vi "merFISH_define_injections_procedure.vi"(0 "Injection procedure IN photobleaching":i32[][](array[numeric]), 1 "Injection procedure IN hybridization":i32[][](array[numeric]), 5 "Buffer Refnum":refnum<vi>, 9 "Start acquisition":bool, 11 "error in":errorcluster, 12 "Defaut injection":i32[][](array[numeric])=[[10, 500, 350, 0], [0, 1200, 120, 0], [10, 500, 300, 21], [5, 2000, 222, 21], [10, 1200, 300, 22], [5, 800, 350, 1], [0, 150, 100, 1]], 13 "Defaut injection photobleaching":i32[][](array[numeric])=[[10, 500, 350, 0], [0, 1200, 120, 0], [10, 500, 300, 21], [5, 2000, 222, 21], [10, 1200, 300, 22], [5, 800, 350, 1], [0, 150, 100, 1]]) -> (3 "Injection procedure OUT":i32[][](array[numeric]), 4 "Injection procedure OUT\nPhotobleaching":i32[][](array[numeric]), 6 "Next task":T1, 10 "error out":errorcluster, 14 "Item Names photobleaching":string[](array[string]), 15 "Item Names":string[](array[string]))   [LabVIEW 2015]
uses:
  CONTROLS/Q_main_element.ctl
panel:
  in  "Default":bool
  in  "Flow rate (µl/min)":i32
  in  "Remove photobleaching":bool
  in  "Select application":i32(ring) caption="Select procedure application" items=["Select procedure application", "HYBRIDIZATION", "PHOTOBLEACHING"]
  in  "Injection procedure PHOTOBLEACHING":i32(listbox)=-1
  in  "Volume (µl)":i32
  in  "Remove":bool
  in  "stop":bool
  in  "Injection procedure HYBRIDIZATION":i32(listbox)=-1
  in  "Add":bool
  in  "Select product":i32(ring) items=["Select product to inject", "ssc", "wb", "ib", "merFISH probe"]
  in  "Pressure (mbar)":i32
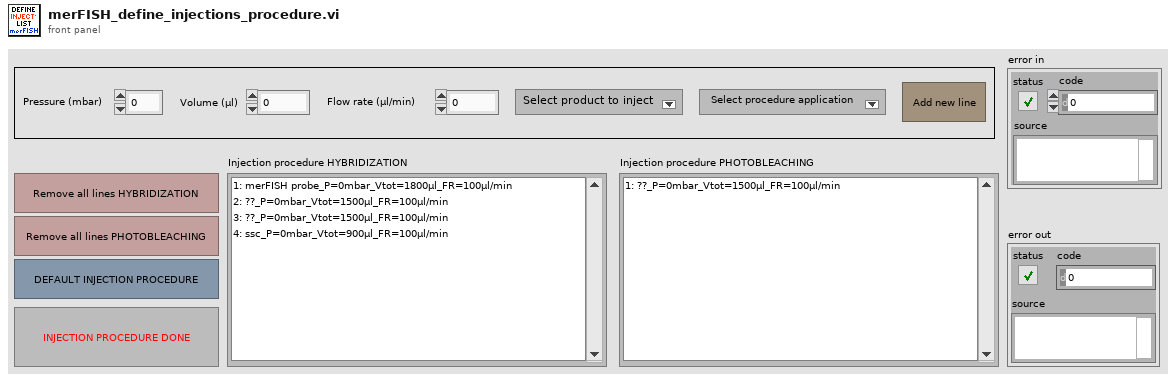
[diagram p1: front panel]
types:
  T1 = typedef "Q_main_element.ctl" = cluster{"variant":variant, "Instruction":enum16{"Main_idle", "Main_initialize", "Main_initialize_TDMS", "Main_initialize_Queue", "Main_error", "Main_DAQ_initialization_results", "Main_ASI_initialization_results", "Main_Piezo_initialization_results", "Main_Valve_initialization_results", "Main_Pump_initialization_results", "Main_CAMERA_initialization_results", "Main_FPGA_initialization_results", "Main_DAQ_error", "Main_ASI_error", "Main_Piezo_error", "Main_CAMERA_error", "Main_Valve_error", "Main_Pump_error", "Main_FPGA_error", "Main_start_acquiring", "Main_not_acquiring", "Main_acquiring", "Main_stop_acquiring", "Main_change_exposure", "Main_change_z_scan_parameters", "Main_define_ROI", "Main_define_mosaic", "Main_read_kinetic_time", "Main_cooler", "Main_read_temperature", "Main_save_XY", "Main_load_XY", "Main_discard_XY", "Main_move_to_XY", "Main_measure_QPD", "Main_autofocus_calibration", "Main_autofocus_initialization", "Main_autofocus_stop", "Main_save_PID", "Main_change_H_valve_position", "Main_two_way_valve", "Main_save_movie", "Main_init_single_scan", "Main_single_scan", "Main_stop_single_scan", "Main_merFISH_illumination_parameters", "Main_merFISH_buffer_probe_list", "Main_merFISH_injections_procedure", "Main_merFISH_save_setpoint", "Main_merFISH_DAPI_parameters", "Main_merFISH_Brightfield_parameters", "Main_merFISH_save_embryo_ROI", "Main_merFISH_init", "Main_merFISH_resume", "Main_merFISH_start_autofocus", "Main_merFISH_open_close_valve_merFISH", "Main_merFISH_open_close_valve_photobleaching", "Main_merFISH_hybridization", "Main_merFISH_move_to_ROI", "Main_merFISH_wait_stabilization", "Main_merFISH_move_to_REF", "Main_merFISH_scan", "Main_merFISH_photobleaching_injection", "Main_merFISH_photobleaching", "Main_merFISH_send_email", "Main_merFISH_close", "Main_STOP"}}
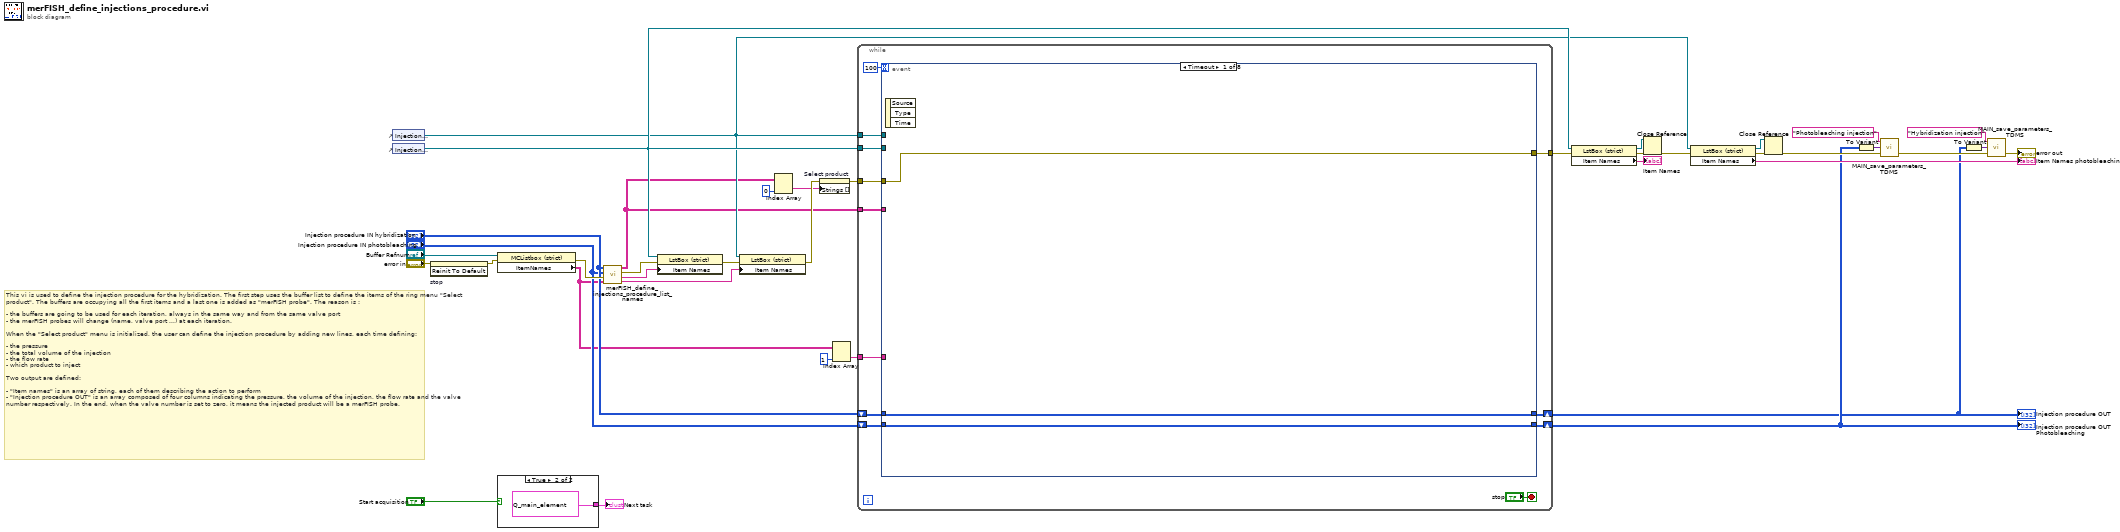
[diagram p0: block diagram]
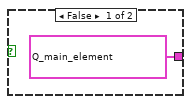
[diagram p2: hidden frame]
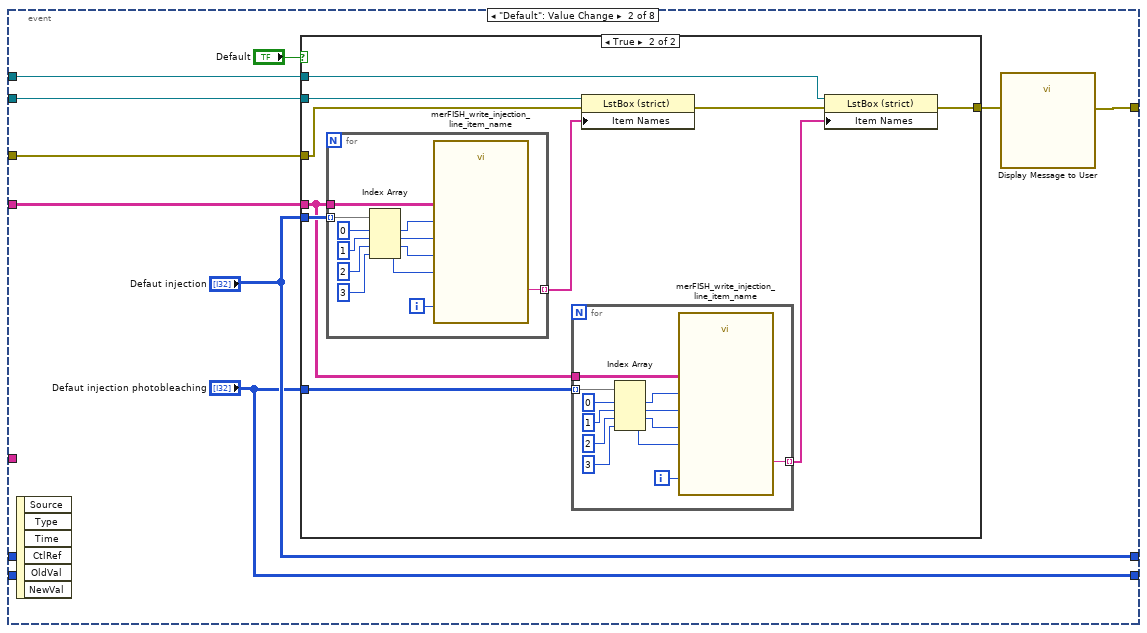
[diagram p3: hidden frame]
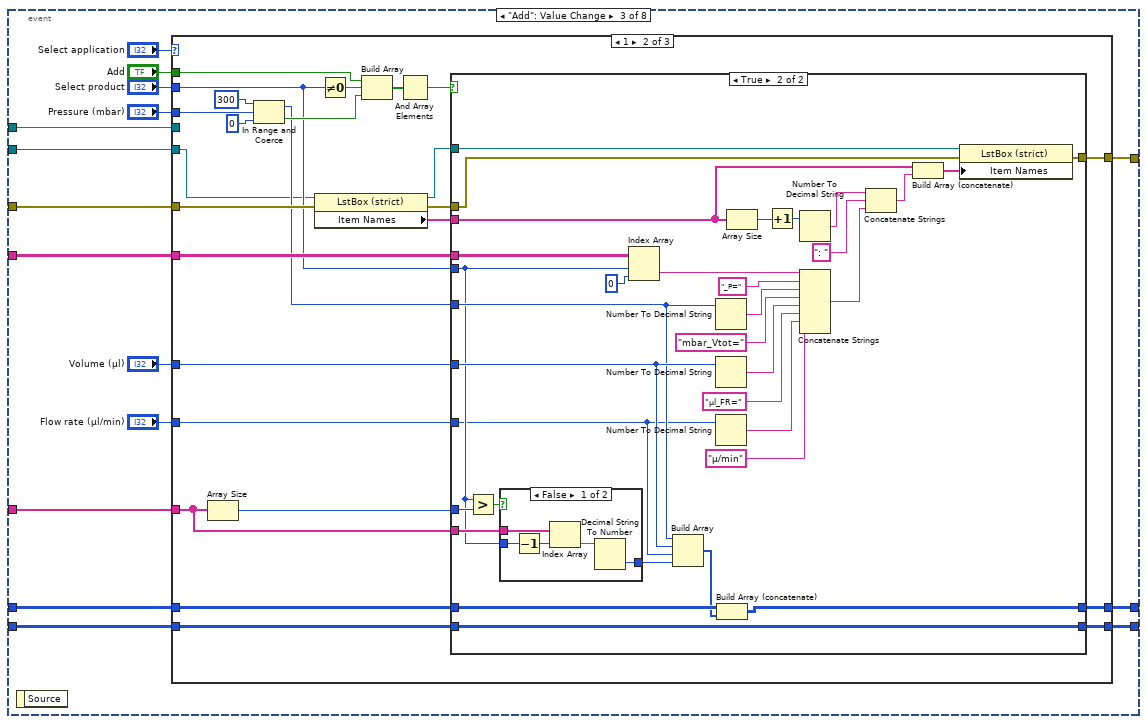
[diagram p5: hidden frame]
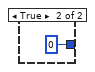
[diagram p8: hidden frame]
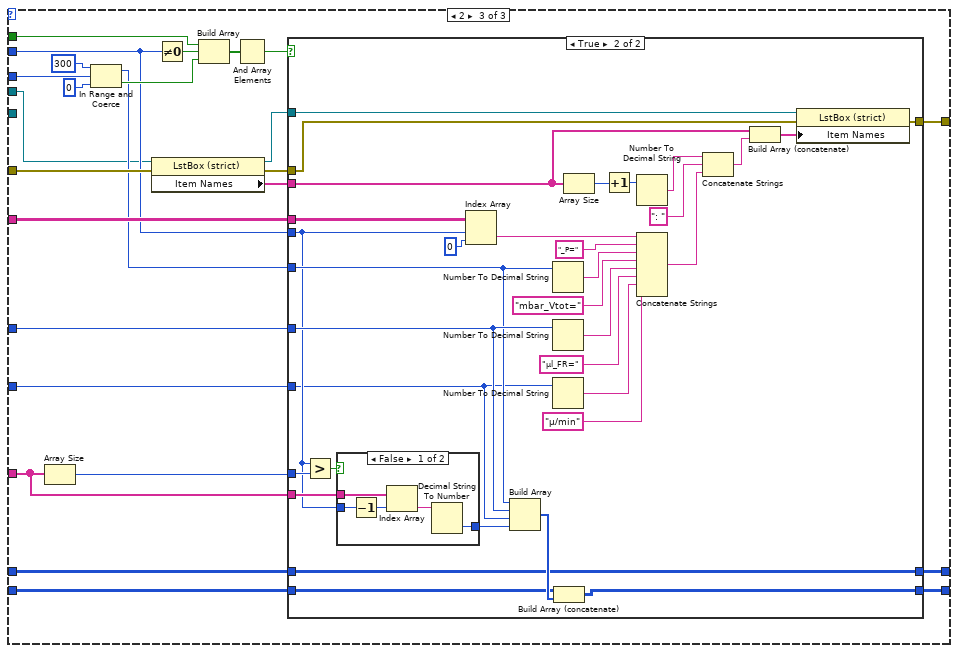
[diagram p9: hidden frame]
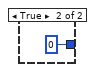
[diagram p11: hidden frame]
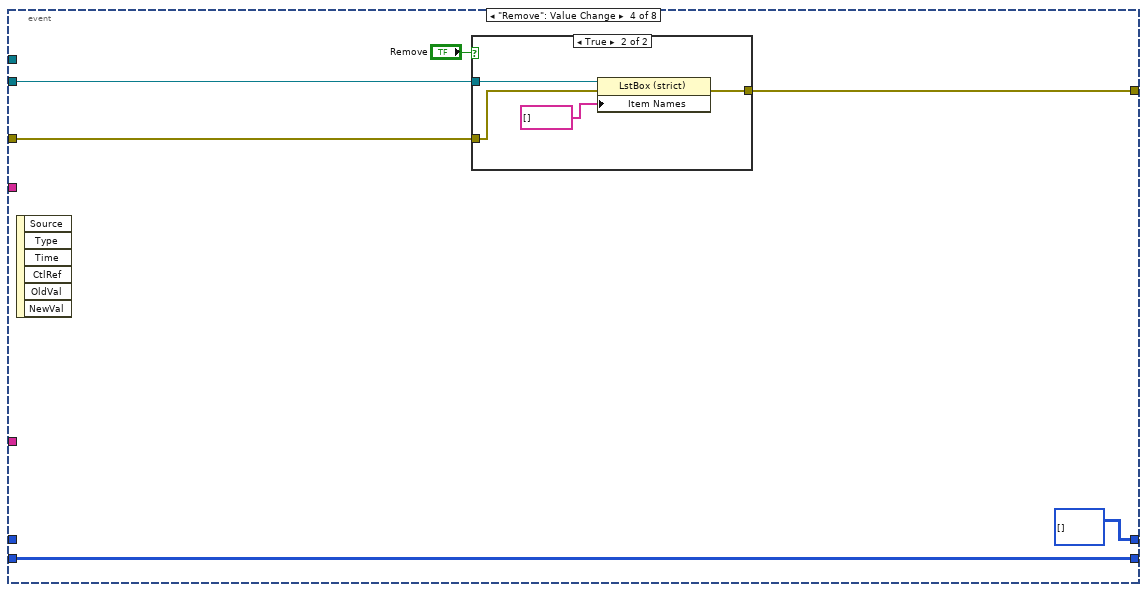
[diagram p12: hidden frame]
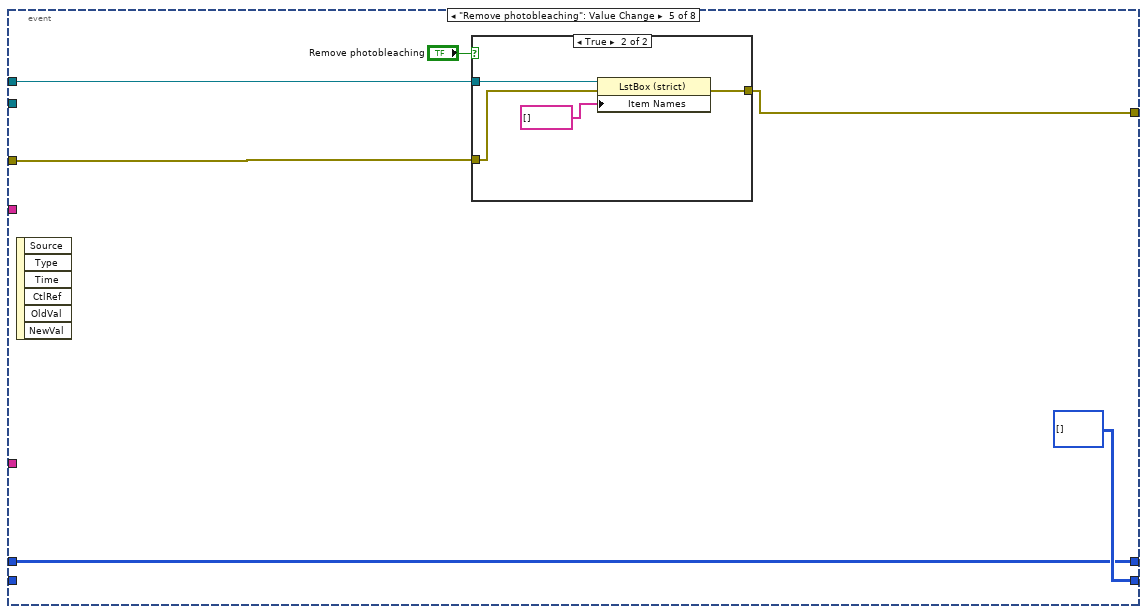
[diagram p14: hidden frame]
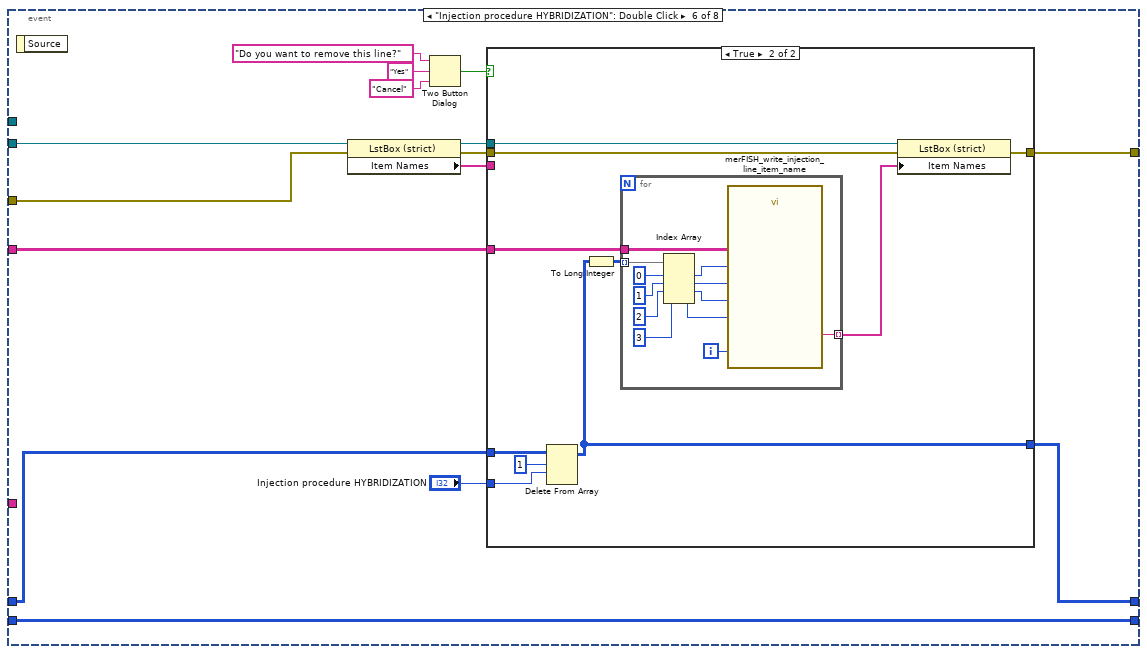
[diagram p16: hidden frame]
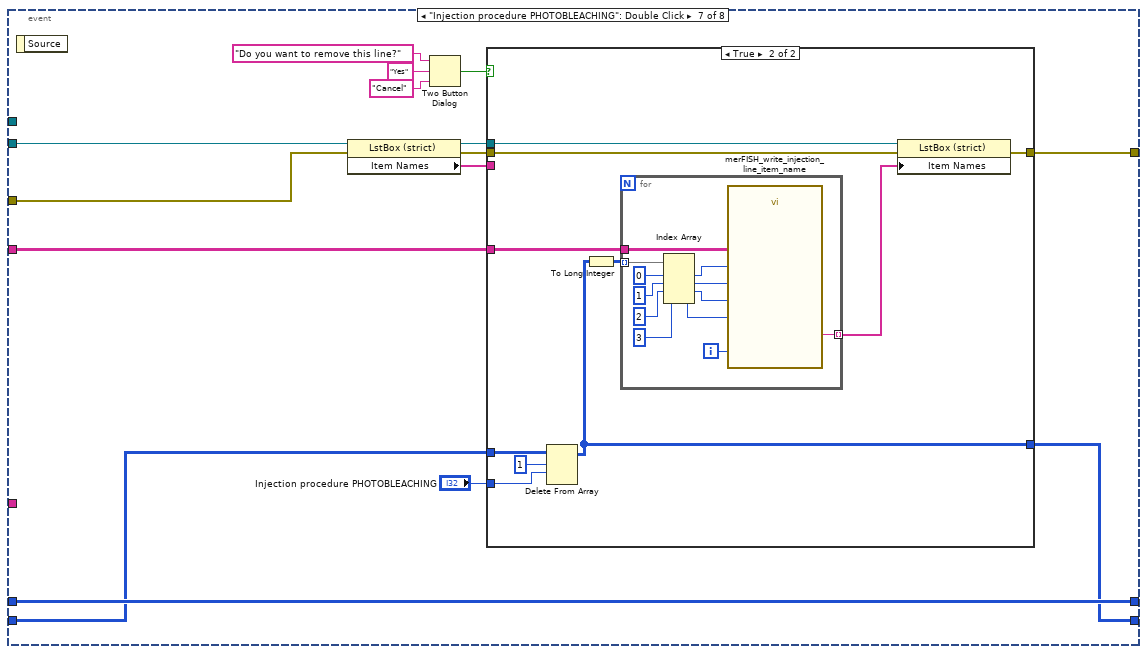
[diagram p18: hidden frame]
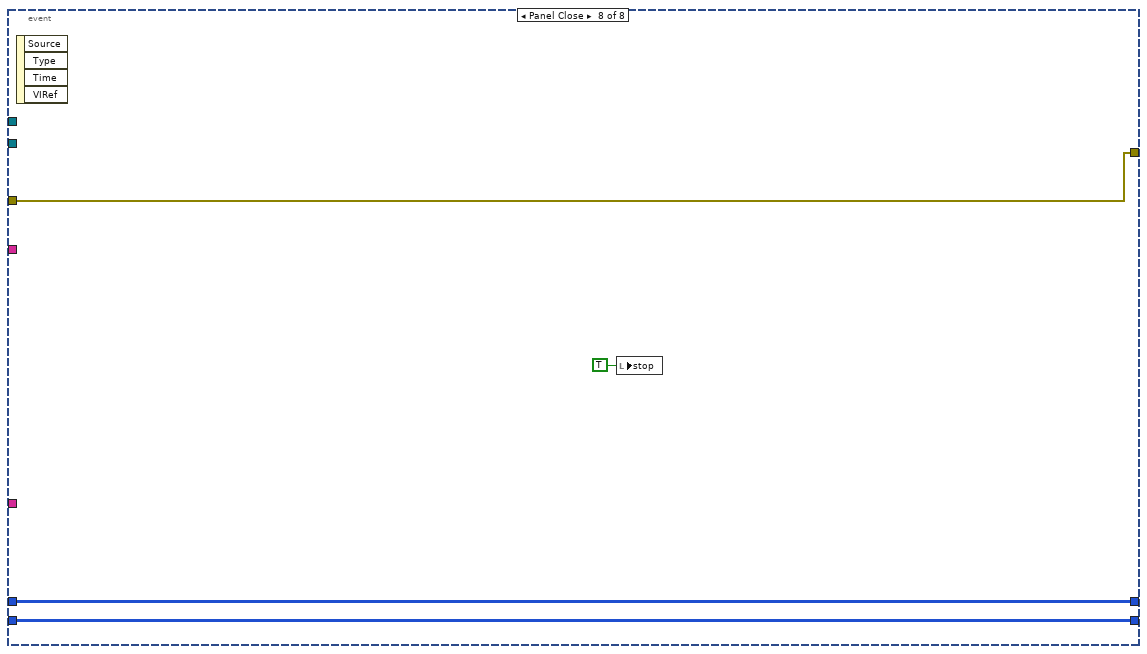
[diagram p20: hidden frame]
diagram:
  # "This vi is used to define the injection procedure for the hybridization. The first step uses the buffer list to define the items of the ring menu \"Select product\". The buffers are occupying all the first items and a last one is added as \"merFISH probe\". The reason is :\n\n- the buffers are going to be used for each iteration, always in the same way and from the same valve port\n- the merFISH probes will change (name, valve port ...) at each iteration.\n\nWhen the \"Select product\" menu is initialized, the user can define the injection procedure by adding new lines, each time defining:\n\n- the pressure\n- the total volume of the injection\n- the flow rate\n- which product to inject\n\nTwo output are defined:\n\n- \"Item names\" is an array of string, each of them describing the action to perform\n- \"Injection procedure OUT\" is an array composed of four columns indicating the pressure, the volume of the injection, the flow rate and the valve number respectively. In the end, when the valve number is set to zero, it means the injected product will be a merFISH probe."
  n1 = control-ref of="Injection procedure PHOTOBLEACHING"() -> (w29:refnum<vi>)
  n2 = control-ref of="Injection manager"() -> (w38:refnum<vi>)
  n3 = invoke on="stop" class="Bool (strict)" method="Reinit To Default"(error in="error in") -> (error out=w1:errorcluster)  [unwired: 2 in, 2 out]
  n4 = property class="MCListbox (strict)"(reference="Buffer Refnum", error in=w1) -> (error out=w28:errorcluster, "ItemNames"=w22:string[][])  [unwired: 1 out]
  n5 = case shown="True" "Start acquisition" {
    tunnel: [T1 {"variant"=variant, "Instruction"=enum."Main_not_acquiring"} ("Q_main_element") T1 {"variant"=variant, "Instruction"=enum."Main_acquiring"} ("Q_main_element")] -> w12
    frame False {
    }
    frame True {
    }
  }
  "Next task" <- w12
  n6 = call "merFISH_define_injections_procedure_list_names.vi"("Buffer list"=w22, "error in"=w28, "Injection procedure IN photobleaching"="Injection procedure IN photobleaching", "Injection procedure IN hybridization"="Injection procedure IN hybridization") -> ("Photobleaching name"=w25:string[], "Hybridization name"=w26:string[], "error out"=w27:errorcluster, "Buffer selection list"=w19:string[][])
  n7 = property class="LstBox (strict)"(reference=w38, error in=w27, "Item Names"=w26) -> (error out=w33:errorcluster)  [unwired: 1 out]
  n8 = property class="LstBox (strict)"(reference=w29, error in=w33, "Item Names"=w25) -> (error out=w32:errorcluster)  [unwired: 1 out]
  n9 = Index Array(array=w19, index (col)=0 ("index (row)")) -> (element=w20:string[])  [unwired: 1 in]
  n10 = property on="Select product" class="Ring (strict)"(error in=w32, "Strings []"=w20) -> (error out=w37:errorcluster)  [unwired: 1 in, 1 out]
  n11 = Index Array(array=w22, index (col)=1 ("disabled index (col)")) -> (element=w34:string[])  [unwired: 1 in]
  n12 = while {
    tunnel: w38 -> [w51]
    tunnel: [w50] -> w39
    tunnel: w19 -> [w49]
    shift-right: [w47] -> w3
    shift-left: "Injection procedure IN hybridization" -> [w48]
    tunnel: w34 -> [w46]
    tunnel: w37 -> [w45]
    tunnel: w29 -> [w44]
    shift-right: [w42] -> w4
    shift-left: "Injection procedure IN photobleaching" -> [w43]
    stop <- "stop" stop-if-true
    n13 = event shown="[0] Timeout" {
      selector: _ -> [_ _ _ _ _ _ _ _]
      dyn-events: _ -> [_ _ _ _ _ _ _ _]
      timeout: 100 -> [_ _ _ _ _ _ _ _]
      tunnel: w51 -> [_ w64 w105 w259 _ w283 w324 _]
      tunnel: w45 -> [w56 w61 w114 w257 w270 w281 w322 w357]
      tunnel: [w56 w62 w116 w256 w269 w286 w325 w357] -> w50
      tunnel: w48 -> [w55 _ w115 _ w265 w285 w317 w356]
      tunnel: w49 -> [_ w65 w113 _ _ w277 w319 _]
      tunnel: [w55 "Defaut injection" w112 i32[][] [] ("Injection procedure IN") w265 w278 w317 w356] -> w47
      tunnel: w46 -> [_ _ w111 _ _ _ _ _]
      tunnel: w44 -> [_ w60 w106 _ w267 _ _ _]
      tunnel: w43 -> [w54 _ w104 w254 _ w276 w316 w355]
      tunnel: [w54 "Defaut injection photobleaching" w103 w254 i32[][] [] ("Injection procedure IN") w276 w315 w355] -> w42
      event Timeout {
        n14 = event-data() -> ()  [unwired: 1 in, 3 out]
      }
      event "Default": Value Change {
        n15 = event-data() -> ()  [unwired: 1 in, 6 out]
        n16 = case shown="True" "Default" {
          tunnel: w65 -> [_ w71]
          tunnel: w64 -> [_ w76]
          tunnel: [w66 w69] -> w63
          tunnel: "Defaut injection" -> [_ w74]
          tunnel: w61 -> [w66 w73]
          tunnel: w60 -> [_ w67]
          tunnel: "Defaut injection photobleaching" -> [_ w72]
          frame False {
          }
          frame True {
            n17 = for {
              tunnel: w74 -> [w99] mode=indexing
              tunnel: [w100] -> w75 mode=indexing
              tunnel: w71 -> [w95]
              i -> [w94]
              n18 = Index Array(array=w99, index #1=0 ("index"), index #2=1 ("index"), index #3=2 ("index"), index #4=3 ("index")) -> (element #1=w93:i32, element #2=w92:i32, element #3=w90:i32, element #4=w89:i32)
              n19 = call "merFISH_write_injection_line_item_name.vi"("Flow rate (µl/min)"=w90, "Select product"=w89, "Injection line number"=w94, "Buffer list"=w95, "Volume (µl)"=w92, "Pressure (mbar)"=w93) -> ("Task name"=w100:string)  [unwired: 3 in]
            }
            n20 = for {
              tunnel: w72 -> [w87] mode=indexing
              tunnel: [w88] -> w68 mode=indexing
              tunnel: w71 -> [w83]
              i -> [w82]
              n21 = Index Array(array=w87, index #1=0 ("index"), index #2=1 ("index"), index #3=2 ("index"), index #4=3 ("index")) -> (element #1=w81:i32, element #2=w80:i32, element #3=w78:i32, element #4=w77:i32)
              n22 = call "merFISH_write_injection_line_item_name.vi"("Flow rate (µl/min)"=w78, "Select product"=w77, "Injection line number"=w82, "Buffer list"=w83, "Volume (µl)"=w80, "Pressure (mbar)"=w81) -> ("Task name"=w88:string)  [unwired: 3 in]
            }
            n23 = property class="LstBox (strict)"(reference=w76, error in=w73, "Item Names"=w75) -> (error out=w70:errorcluster)  [unwired: 1 out]
            n24 = property class="LstBox (strict)"(reference=w67, error in=w70, "Item Names"=w68) -> (error out=w69:errorcluster)  [unwired: 1 out]
          }
        }
        n25 = call "Display Message to User"("error in (no error)"=w63) -> ("error out"=w62:errorcluster)  [unwired: 9 in, 1 out]
      }
      event "Add": Value Change {
        n26 = event-data() -> ()  [unwired: 1 in, 1 out]
        n27 = case shown="1" "Select application" {
          tunnel: [w118 w144 w211] -> w116
          tunnel: w115 -> [w119 w143 w210]
          tunnel: w114 -> [w118 w142 w209]
          tunnel: w113 -> [_ w132 w199]
          tunnel: [w119 w130 w197] -> w112
          tunnel: w111 -> [_ w128 w195]
          tunnel: "Add" -> [_ w127 w194]
          tunnel: "Select product" -> [_ w126 w193]
          tunnel: "Pressure (mbar)" -> [_ w125 w192]
          tunnel: w106 -> [_ _ w187]
          tunnel: w105 -> [_ w124 _]
          tunnel: w104 -> [w117 w123 w191]
          tunnel: [w117 w122 w190] -> w103
          tunnel: "Volume (µl)" -> [_ w121 w189]
          tunnel: "Flow rate (µl/min)" -> [_ w120 w188]
          frame 0, Default {
          }
          frame 1 {
            n28 = Array Size(array=w128) -> (size(s)=w129:i32)
            n29 = In Range and Coerce(upper limit=300, x=w125, lower limit=0) -> (coerced(x)=w131:i32, In Range?=w133:bool)
            n30 = property class="LstBox (strict)"(reference=w124, error in=w142) -> (reference out=w137:refnum<vi>, error out=w138:errorcluster, "Item Names"=w136:string[])
            n31 = Not Equal To 0?(x=w126) -> (x != 0?=w141:bool)
            n32 = Build Array(w127, w141, w133) -> (w140:bool[])
            n33 = And Array Elements(Boolean array=w140) -> (logical AND=w139:bool)
            n34 = case shown="True" w139 {
              tunnel: w137 -> [_ w177]
              tunnel: w126 -> [_ w156]
              tunnel: [w147 w173] -> w144
              tunnel: w138 -> [w147 w168]
              tunnel: w143 -> [w146 w172]
              tunnel: [w146 w171] -> w130
              tunnel: w136 -> [_ w169]
              tunnel: w121 -> [_ w161]
              tunnel: w132 -> [_ w167]
              tunnel: w131 -> [_ w159]
              tunnel: w129 -> [_ w158]
              tunnel: w128 -> [_ w157]
              tunnel: w123 -> [w145 w153]
              tunnel: [w145 w153] -> w122
              tunnel: w120 -> [_ w150]
              frame False {
              }
              frame True {
                n35 = Greater?(x=w156, y=w158) -> (0:w154:bool)
                n36 = case shown="False" w154 {
                  tunnel: w157 -> [w185 _]
                  tunnel: w156 -> [w184 _]
                  tunnel: [w181 0] -> w149
                  frame False {
                    n37 = Decrement(x=w184) -> (x-1=w183:i32)
                    n38 = Index Array(array=w185, index=w183) -> (element=w182:string)
                    n39 = Decimal String To Number(string=w182) -> (number=w181:i32)  [unwired: 2 in, 1 out]
                  }
                  frame True {
                  }
                }
                n40 = Index Array(array=w167, index (row)=w156, index (col)=0 ("disabled index (col)")) -> (element=w166:string)
                n41 = Build Array(w159, w161, w150, w149) -> (w155:i32[])
                n42 = Number To Decimal String(number=w159) -> (decimal integer string=w164:string)  [unwired: 1 in]
                n43 = Number To Decimal String(number=w161) -> (decimal integer string=w162:string)  [unwired: 1 in]
                n44 = Number To Decimal String(number=w150) -> (decimal integer string=w152:string)  [unwired: 1 in]
                n45 = Build Array (concatenate)(w172, w155) -> (w171:i32[][])
                n46 = Array Size(array=w169) -> (size(s)=w176:i32)
                n47 = Increment(x=w176) -> (x+1=w180:i32)
                n48 = Number To Decimal String(number=w180) -> (decimal integer string=w179:string)  [unwired: 1 in]
                n49 = Concatenate Strings(w166, "_P=" ("string"), w164, "mbar_Vtot=" ("string"), w162, "µl_FR=" ("string"), w152, "µ/min" ("string")) -> (w174:string)
                n50 = Concatenate Strings(w179, ": " ("string"), w174) -> (w178:string)
                n51 = Build Array (concatenate)(w169, w178) -> (w170:string[])
                n52 = property class="LstBox (strict)"(reference=w177, error in=w168, "Item Names"=w170) -> (error out=w173:errorcluster)  [unwired: 1 out]
              }
            }
          }
          frame 2 {
            n53 = Array Size(array=w195) -> (size(s)=w196:i32)
            n54 = In Range and Coerce(upper limit=300, x=w192, lower limit=0) -> (coerced(x)=w198:i32, In Range?=w200:bool)
            n55 = property class="LstBox (strict)"(reference=w187, error in=w209) -> (reference out=w204:refnum<vi>, error out=w205:errorcluster, "Item Names"=w203:string[])
            n56 = Not Equal To 0?(x=w193) -> (x != 0?=w208:bool)
            n57 = Build Array(w194, w208, w200) -> (w207:bool[])
            n58 = And Array Elements(Boolean array=w207) -> (logical AND=w206:bool)
            n59 = case shown="True" w206 {
              tunnel: w204 -> [_ w244]
              tunnel: w193 -> [_ w225]
              tunnel: [w214 w240] -> w211
              tunnel: w205 -> [w214 w237]
              tunnel: w210 -> [w213 w217]
              tunnel: [w213 w217] -> w197
              tunnel: w203 -> [_ w238]
              tunnel: w189 -> [_ w230]
              tunnel: w199 -> [_ w236]
              tunnel: w198 -> [_ w228]
              tunnel: w196 -> [_ w227]
              tunnel: w195 -> [_ w226]
              tunnel: w191 -> [w212 w218]
              tunnel: [w212 w216] -> w190
              tunnel: w188 -> [_ w220]
              frame False {
              }
              frame True {
                n60 = Greater?(x=w225, y=w227) -> (0:w223:bool)
                n61 = case shown="False" w223 {
                  tunnel: w226 -> [w252 _]
                  tunnel: w225 -> [w251 _]
                  tunnel: [w248 0] -> w219
                  frame False {
                    n62 = Decrement(x=w251) -> (x-1=w250:i32)
                    n63 = Index Array(array=w252, index=w250) -> (element=w249:string)
                    n64 = Decimal String To Number(string=w249) -> (number=w248:i32)  [unwired: 2 in, 1 out]
                  }
                  frame True {
                  }
                }
                n65 = Index Array(array=w236, index (row)=w225, index (col)=0 ("disabled index (col)")) -> (element=w235:string)
                n66 = Build Array(w228, w230, w220, w219) -> (w224:i32[])
                n67 = Number To Decimal String(number=w228) -> (decimal integer string=w233:string)  [unwired: 1 in]
                n68 = Number To Decimal String(number=w230) -> (decimal integer string=w231:string)  [unwired: 1 in]
                n69 = Number To Decimal String(number=w220) -> (decimal integer string=w222:string)  [unwired: 1 in]
                n70 = Build Array (concatenate)(w218, w224) -> (w216:i32[][])
                n71 = Array Size(array=w238) -> (size(s)=w243:i32)
                n72 = Increment(x=w243) -> (x+1=w247:i32)
                n73 = Number To Decimal String(number=w247) -> (decimal integer string=w246:string)  [unwired: 1 in]
                n74 = Concatenate Strings(w235, "_P=" ("string"), w233, "mbar_Vtot=" ("string"), w231, "µl_FR=" ("string"), w222, "µ/min" ("string")) -> (w241:string)
                n75 = Concatenate Strings(w246, ": " ("string"), w241) -> (w245:string)
                n76 = Build Array (concatenate)(w238, w245) -> (w239:string[])
                n77 = property class="LstBox (strict)"(reference=w244, error in=w237, "Item Names"=w239) -> (error out=w240:errorcluster)  [unwired: 1 out]
              }
            }
          }
        }
      }
      event "Remove": Value Change {
        n78 = event-data() -> ()  [unwired: 1 in, 6 out]
        n79 = case shown="True" "Remove" {
          tunnel: w259 -> [_ w264]
          tunnel: w257 -> [w260 w263]
          tunnel: [w260 w262] -> w256
          frame False {
          }
          frame True {
            n80 = property class="LstBox (strict)"(reference=w264, error in=w263, "Item Names"=string[] []) -> (error out=w262:errorcluster)  [unwired: 1 out]
          }
        }
      }
      event "Remove photobleaching": Value Change {
        n81 = event-data() -> ()  [unwired: 1 in, 6 out]
        n82 = case shown="True" "Remove photobleaching" {
          tunnel: w267 -> [_ w275]
          tunnel: w270 -> [w271 w274]
          tunnel: [w271 w273] -> w269
          frame False {
          }
          frame True {
            n83 = property class="LstBox (strict)"(reference=w275, error in=w274, "Item Names"=string[] []) -> (error out=w273:errorcluster)  [unwired: 1 out]
          }
        }
      }
      event "Injection procedure HYBRIDIZATION": Double Click {
        n84 = event-data() -> ()  [unwired: 1 in, 1 out]
        n85 = property class="LstBox (strict)"(reference=w283, error in=w281) -> (reference out=w282:refnum<vi>, error out=w280:errorcluster, "Item Names"=w279:string[])
        n86 = Two Button Dialog(message="Do you want to remove this line?", 1:"Cancel" ("F button name (\"Cancel\")"), 2:"Yes" ("T button name (\"OK\")")) -> (T button?=w287:bool)
        n87 = case shown="True" w287 {
          tunnel: w282 -> [_ w297]
          tunnel: [w291 w302] -> w286
          tunnel: w285 -> [w292 w301]
          tunnel: [w292 w295] -> w278
          tunnel: "Injection procedure HYBRIDIZATION" -> [_ w299]
          tunnel: w280 -> [w291 w298]
          tunnel: w279 -> [_ _]
          tunnel: w277 -> [_ w293]
          frame False {
          }
          frame True {
            n88 = Delete From Array(array=w301, length=1, index (row)=w299) -> (array with subset deleted=w295:i32[][])  [unwired: 1 in, 1 out]
            n89 = To Long Integer(number=w295) -> (32bit integer=w294:i32[][])
            n90 = for {
              tunnel: w294 -> [w313] mode=indexing
              tunnel: [w314] -> w296 mode=indexing
              tunnel: w293 -> [w309]
              i -> [w308]
              n91 = Index Array(array=w313, index #1=0 ("index"), index #2=1 ("index"), index #3=2 ("index"), index #4=3 ("index")) -> (element #1=w307:i32, element #2=w306:i32, element #3=w304:i32, element #4=w303:i32)
              n92 = call "merFISH_write_injection_line_item_name.vi"("Flow rate (µl/min)"=w304, "Select product"=w303, "Injection line number"=w308, "Buffer list"=w309, "Volume (µl)"=w306, "Pressure (mbar)"=w307) -> ("Task name"=w314:string)  [unwired: 3 in]
            }
            n93 = property class="LstBox (strict)"(reference=w297, error in=w298, "Item Names"=w296) -> (error out=w302:errorcluster)  [unwired: 1 out]
          }
        }
      }
      event "Injection procedure PHOTOBLEACHING": Double Click {
        n94 = event-data() -> ()  [unwired: 1 in, 1 out]
        n95 = property class="LstBox (strict)"(reference=w324, error in=w322) -> (reference out=w323:refnum<vi>, error out=w321:errorcluster, "Item Names"=w320:string[])
        n96 = Two Button Dialog(message="Do you want to remove this line?", 1:"Cancel" ("F button name (\"Cancel\")"), 2:"Yes" ("T button name (\"OK\")")) -> (T button?=w326:bool)
        n97 = case shown="True" w326 {
          tunnel: w323 -> [_ w336]
          tunnel: [w330 w341] -> w325
          tunnel: w316 -> [w331 w340]
          tunnel: [w331 w334] -> w315
          tunnel: "Injection procedure PHOTOBLEACHING" -> [_ w338]
          tunnel: w321 -> [w330 w337]
          tunnel: w320 -> [_ _]
          tunnel: w319 -> [_ w332]
          frame False {
          }
          frame True {
            n98 = Delete From Array(array=w340, length=1, index (row)=w338) -> (array with subset deleted=w334:i32[][])  [unwired: 1 in, 1 out]
            n99 = To Long Integer(number=w334) -> (32bit integer=w333:i32[][])
            n100 = for {
              tunnel: w333 -> [w352] mode=indexing
              tunnel: [w353] -> w335 mode=indexing
              tunnel: w332 -> [w348]
              i -> [w347]
              n101 = Index Array(array=w352, index #1=0 ("index"), index #2=1 ("index"), index #3=2 ("index"), index #4=3 ("index")) -> (element #1=w346:i32, element #2=w345:i32, element #3=w343:i32, element #4=w342:i32)
              n102 = call "merFISH_write_injection_line_item_name.vi"("Flow rate (µl/min)"=w343, "Select product"=w342, "Injection line number"=w347, "Buffer list"=w348, "Volume (µl)"=w345, "Pressure (mbar)"=w346) -> ("Task name"=w353:string)  [unwired: 3 in]
            }
            n103 = property class="LstBox (strict)"(reference=w336, error in=w337, "Item Names"=w335) -> (error out=w341:errorcluster)  [unwired: 1 out]
          }
        }
      }
      event Panel Close {
        n104 = event-data() -> ()  [unwired: 1 in, 4 out]
        n105 = local write "stop"(TRUE ("stop")) -> ()
      }
    }
  }
  "Injection procedure OUT" <- w3
  "Injection procedure OUT\nPhotobleaching" <- w4
  n106 = property class="LstBox (strict)"(reference=w38, error in=w39) -> (reference out=w18:refnum<vi>, error out=w17:errorcluster, "Item Names"=→"Item Names":string[])
  n107 = Close Reference(reference=w18, error in (no error)=w17) -> (error out=w16:errorcluster)
  n108 = property class="LstBox (strict)"(reference=w29, error in=w16) -> (reference out=w14:refnum<vi>, error out=w15:errorcluster, "Item Names"=→"Item Names photobleaching":string[])
  n109 = Close Reference(reference=w14, error in (no error)=w15) -> (error out=w7:errorcluster)
  n110 = To Variant(anything=w4) -> (Variant=w8:variant)
  n111 = call "MAIN_save_parameters_TDMS.vi"("error in"=w7, "Data"=w8, "Channel name"="Photobleaching injection" ("group name")) -> ("error out"=w5:errorcluster)  [unwired: 2 in]
  n112 = To Variant(anything=w3) -> (Variant=w11:variant)
  n113 = call "MAIN_save_parameters_TDMS.vi"("error in"=w5, "Data"=w11, "Channel name"="Hybridization injection" ("group name")) -> ("error out"=→"error out":errorcluster)  [unwired: 2 in]
